vi "JSONRPC-GetMethodInfo.vi"(8 "error in":errorcluster, 11 "input string":string) -> (0 "error out":errorcluster, 2 "RPC":T1={"params"="", "id"="", "method"=enum."UNDEFINED"}, 3 "input string":string)   [LabVIEW 2014]
doc: "Searches <b>input string</b> for a JSONRPC 2.0 call. If found, <b>RPC</b> contains the ID, method and params of the call."
panel:
  in  "output cluster":T1={"params"="", "id"="", "method"=enum."UNDEFINED"}
  # "JSONRPC-GetMethodInfo"
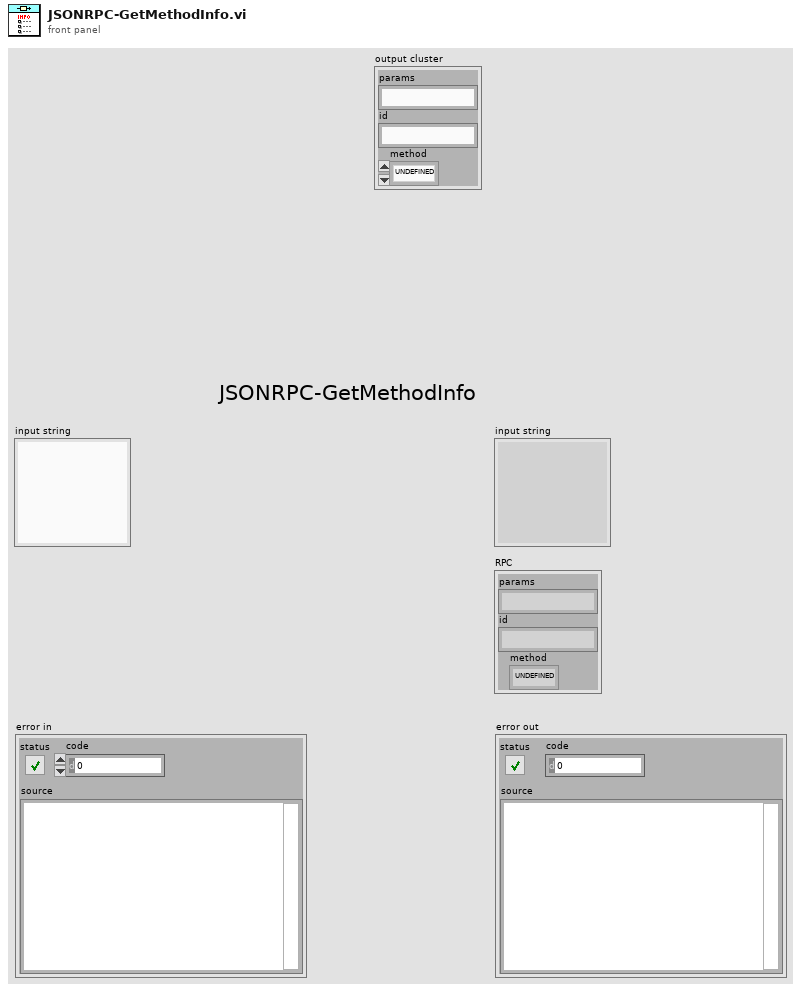
[diagram p1: front panel]
types:
  T1 = cluster{"params":string, "id":string, "method":enum16{"open", "close", "start", "stop", "get", "set", "info", "UNDEFINED"}}
  T2 = enum16{"open", "close", "start", "stop", "get", "set", "info", "UNDEFINED"}
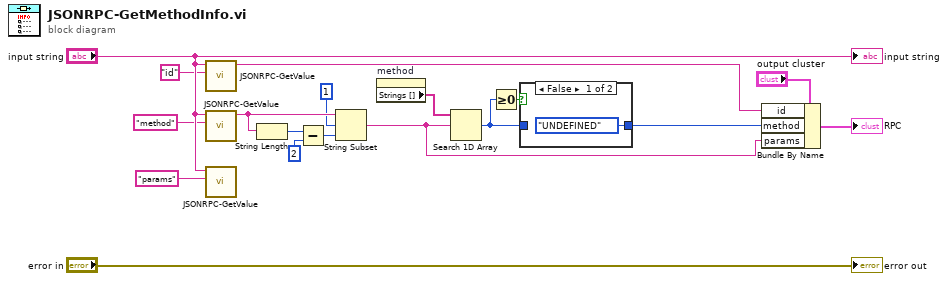
[diagram p0: block diagram]
diagram:
  n1 = call "JSONRPC-GetValue.vi"("key"="id" ("Key"), "input string"="input string") -> ("value"=w13:string)  [unwired: 9 in]
  n2 = call "JSONRPC-GetValue.vi"("key"="method" ("Key"), "input string"="input string") -> ("value"=w11:string)  [unwired: 9 in]
  n3 = call "JSONRPC-GetValue.vi"("key"="params" ("Key"), "input string"="input string") -> ()  [unwired: 9 in, 1 out]
  n4 = String Length(string=w11) -> (length=w9:i32)
  n5 = Subtract(x=w9, y=2) -> (x-y=w7:i32)
  n6 = String Subset(string=w11, offset (0)=1, length (rest)=w7) -> (substring=w2:string)
  n7 = property on="method" class="Enum (strict)"() -> ("Strings []"=w4:string[])  [unwired: 2 in, 2 out]
  n8 = Search 1D Array(1D array=w4, element=w2) -> (index of element=w5:i32)  [unwired: 1 in]
  n9 = Greater Or Equal To 0?(x=w5) -> (x >= 0?=w17:bool)
  n10 = case shown="False" w17 {
    tunnel: [T2."UNDEFINED" ("method") w20] -> w3
    tunnel: w5 -> [_ w20]
    frame False {
    }
    frame True {
    }
  }
  n11 = Bundle By Name(cluster="output cluster", "id"=w13, "method"=w3, "params"=w2) -> (→"RPC":T1)
  "error out" <- "error in"
  "input string" <- "input string"
